vi "Determine Output Value.vi"(10 "Output Segments":string="cdfeb fcadb cdfeb cdbaf", 11 "Digit Patterns":cluster{i32[]}[](array[cluster])=[{[0, 1, 2, 3, 4, 5]}, {[0, 1]}, {[0, 2, 3, 5, 6]}, {[0, 1, 2, 3, 5]}, {[0, 1, 4, 5]}, {[1, 2, 3, 4, 5]}, {[1, 2, 3, 4, 5, 6]}, {[0, 1, 3]}, {[0, 1, 2, 3, 4, 5, 6]}, {[0, 1, 2, 3, 4, 6]}]) -> (3 "Output Value":i32)   [LabVIEW 2020]
panel:
  out "Digits":i32[](array[numeric])
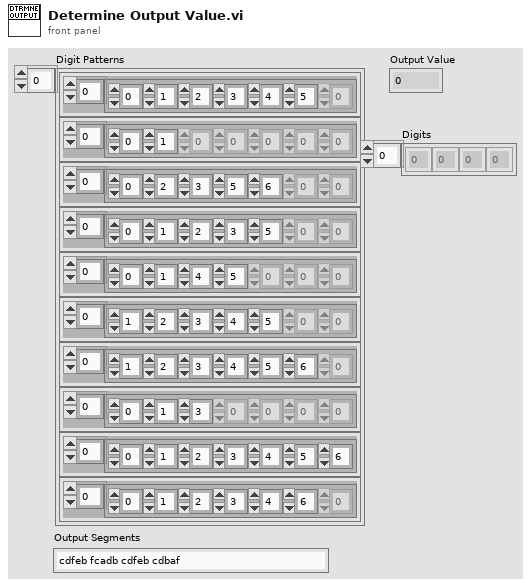
[diagram p1: front panel]
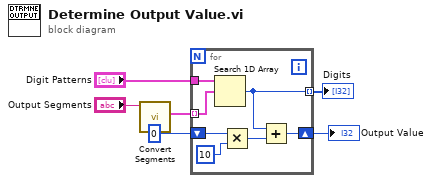
[diagram p0: block diagram]
diagram:
  n1 = call "Convert Segments.vi"("Pattern String"="Output Segments") -> ("Segment Indices"=w4:cluster{i32[]}[])  [unwired: 9 in, 1 out]
  n2 = for {
    tunnel: "Digit Patterns" -> [w13]
    tunnel: w4 -> [w12] mode=indexing
    shift-right: [w8] -> w2
    shift-left: 0 -> [w11]
    tunnel: [w7] -> w1 mode=indexing
    n3 = Search 1D Array(1D array=w13, element=w12) -> (index of element=w7:i32)  [unwired: 1 in]
    n4 = Multiply(x=w11, y=10) -> (x*y=w9:i32)
    n5 = Add(x=w7, y=w9) -> (x+y=w8:i32)
  }
  "Output Value" <- w2
  "Digits" <- w1
